vi "Parse_array_string_settings.vi"(8 "error in (no error)":errorcluster, 11 "Value":string) -> (0 "error out":errorcluster, 3 "Output":string[](array[string]))   [LabVIEW 2020, in "Config.lvclass"]
uses:
  Config/Config.lvclass
  <vilib>/regexp/Match Regular Expression.xnode
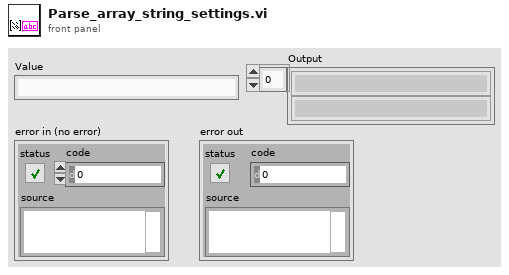
[diagram p1: front panel]
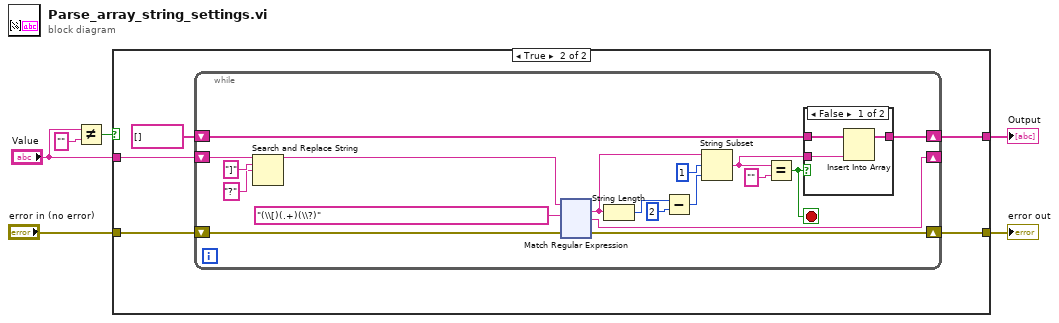
[diagram p0: block diagram]
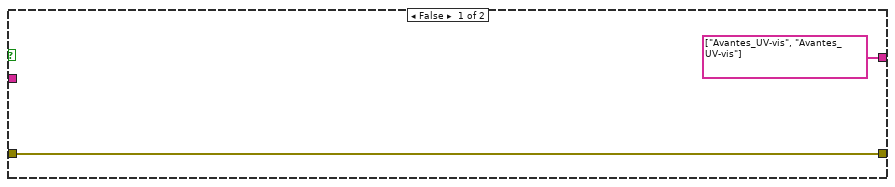
[diagram p2: hidden frame]
diagram:
  n1 = Not Equal?(x="Value", y="") -> (x != y?=w3:bool)
  n2 = case shown="True" w3 {
    tunnel: "error in (no error)" -> [w8 w13]
    tunnel: [w8 w12] -> w5
    tunnel: "Value" -> [_ w11]
    tunnel: [string[] ["Avantes_UV-vis", "Avantes_UV-vis"] ("Array 2") w10] -> w1
    frame False {
    }
    frame True {
      n3 = while {
        shift-right: [w31] -> _
        shift-left: w11 -> [w23]
        shift-right: [w27] -> w10
        shift-left: string[] [] ("Array 2") -> [w26]
        shift-right: [w24] -> w12
        shift-left: w13 -> [w25]
        stop <- w28 stop-if-true
        n4 = Search and Replace String(input string=w23, search string="]", replace string="?" ("replace string (\"\")")) -> (result string=w20:string)  [unwired: 5 in, 3 out]
        n5 = xnode "Match Regular Expression"("input string"=w20, "regular expression"="(\\[)(.+)(\\?)", "error in"=w25) -> ("whole match"=w14:string, "after match"=w31:string, "error out"=w24:errorcluster)  [unwired: 3 in, 2 out]
        n6 = String Length(string=w14) -> (length=w17:i32)
        n7 = Subtract(x=w17, y=2) -> (x-y=w15:i32)
        n8 = String Subset(string=w14, offset (0)=1, length (rest)=w15) -> (substring=w19:string)
        n9 = Equal?(x=w19, y="") -> (x = y?=w28:bool)
        n10 = case shown="False" w28 {
          tunnel: w19 -> [w32 _]
          tunnel: [w33 w35] -> w27
          tunnel: w26 -> [w34 w35]
          frame False {
            n11 = Insert Into Array(array=w34, new element=w32) -> (w33:string[])  [unwired: 1 in]
          }
          frame True {
          }
        }
      }
    }
  }
  "error out" <- w5
  "Output" <- w1
